vi "WriteLog.vi"(8 "error in (no error)":errorcluster caption="错误输入（无错误）", 9 "Model":string, 10 "Type":enum16{"一般日志", "警告日志", "错误日志", "致命日志", "一场日志"}(ring), 11 "MSG":string) -> (0 "错误输出":errorcluster)   [LabVIEW 2018]
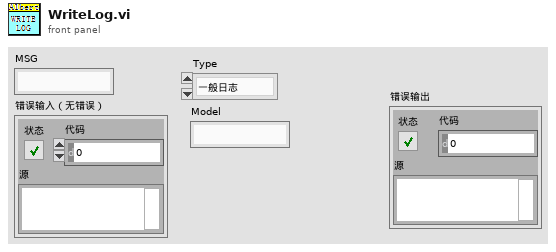
[diagram p1: front panel]
types:
  T1 = enum16{"open", "replace", "create", "open or create", "replace or create", "replace or create with confirmation"}
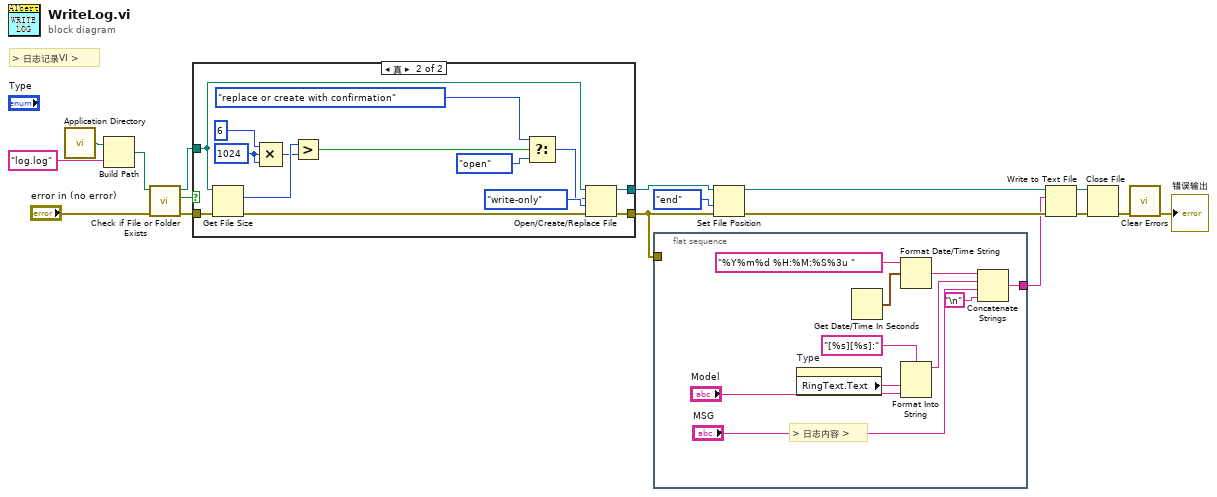
[diagram p0: block diagram]
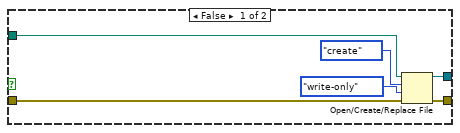
[diagram p2: hidden frame]
diagram:
  # "> 日志记录VI >"
  n1 = call <vilib>:"Application Directory.vi"() -> ("Application Directory"=w13:path)
  n2 = Build Path(base path=w13, name or relative path="log.log") -> (appended path=w11:path)
  n3 = call <vilib>:"Check if File or Folder Exists.vi"("error in (no error)"="error in (no error)", "path"=w11) -> ("error out"=w8:errorcluster, "file or folder exists?"=w10:bool, "dup path"=w9:path)  [unwired: 7 in]
  n4 = case shown="真" w10 {
    tunnel: w9 -> [w21 w29]
    tunnel: w8 -> [w20 w37]
    tunnel: [w18 w26] -> w6
    tunnel: [w19 w25] -> w5
    frame False {
      n5 = Open/Create/Replace File(file path (use dialog)=w21, error in=w20, operation (0:open)=T1."create" ("操作(0:open)"), access (0:read/write)=enum16{"read/write", "read-only", "write-only"}."write-only" ("权限(0:read/write)")) -> (refnum out=w19:refnum<file>, error out=w18:errorcluster)  [unwired: 2 in, 1 out]
    }
    frame True {
      w34 = 1024 ("值")
      n6 = Get File Size(file=w29, error in=w37) -> (size (in bytes)=w36:i64, 0:w27:errorcluster)  [unwired: 1 out]
      n7 = Compound Arithmetic op=MULTIPLY(6, w34, w34) -> (w24:i32)
      n8 = Greater?(x=w36, y=w24) -> (0:w32:bool)
      n9 = Select(t=T1."replace or create with confirmation" ("操作(0:open)"), s=w32, f=T1."open" ("操作(0:open)")) -> (s? t:f=w28:T1)
      n10 = Open/Create/Replace File(file path (use dialog)=w29, error in=w27, operation (0:open)=w28, access (0:read/write)=enum16{"read/write", "read-only", "write-only"}."write-only" ("权限(0:read/write)")) -> (refnum out=w25:refnum<file>, error out=w26:errorcluster)  [unwired: 2 in, 1 out]
    }
  }
  n11 = flat-sequence {
    tunnel: [w44] -> w14
    tunnel: w6 -> [_]
    frame #0 {
      # "> 日志内容 >"
      n12 = property on="Type" class="Enum (严格)"() -> ("RingText.Text"=w38:string)  [unwired: 2 in, 2 out]
      n13 = Get Date/Time In Seconds() -> (seconds since 1Jan1904=w47:timestamp)
      n14 = Format Date/Time String(time format string (%c)="%Y%m%d %H:%M:%S%3u " ("时间格式字符串(%c)"), seconds (now)=w47) -> (date/time string=w45:string)  [unwired: 1 in]
      n15 = Format Into String(format string="[%s][%s]:" ("格式字符串"), w38, "Model") -> (resulting string=w41:string)  [unwired: 2 in, 1 out]
      n16 = Concatenate Strings(w45, w41, "MSG", "\n") -> (w44:string)
    }
  }
  n17 = Set File Position(refnum=w5, from (0:start)=enum16{"start", "end", "current"}."end" ("自（0:起始）"), error in=w6) -> (refnum out=w16:refnum<file>, error out=w15:errorcluster)  [unwired: 1 in]
  n18 = Write to Text File(file (use dialog)=w16, text=w14, error in=w15) -> (refnum out=w3:refnum<file>, error out=w4:errorcluster)  [unwired: 1 in, 1 out]
  n19 = Close File(refnum=w3, error in=w4) -> (error out=w2:errorcluster)  [unwired: 1 out]
  n20 = call <vilib>:"Clear Errors.vi"("error in (no error)"=w2) -> ("error out"=→"错误输出":errorcluster)  [unwired: 5 in, 1 out]
